vi "criocon.vi"() -> ()   [LabVIEW 2017]
panel:
  in  "Tab Control":enum32{"Page 1", "Page 2"}(tab)
  out "T (K)":dbl=20.57397 format="%6.3f"
  in  "stop":bool
  in  "VISA Resource Name":refnum<visa-resource-name>="GPIB0::12::INSTR"
  in  "wait (ms)":u32=20
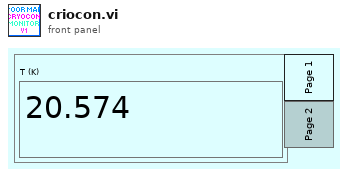
[diagram p1: front panel]
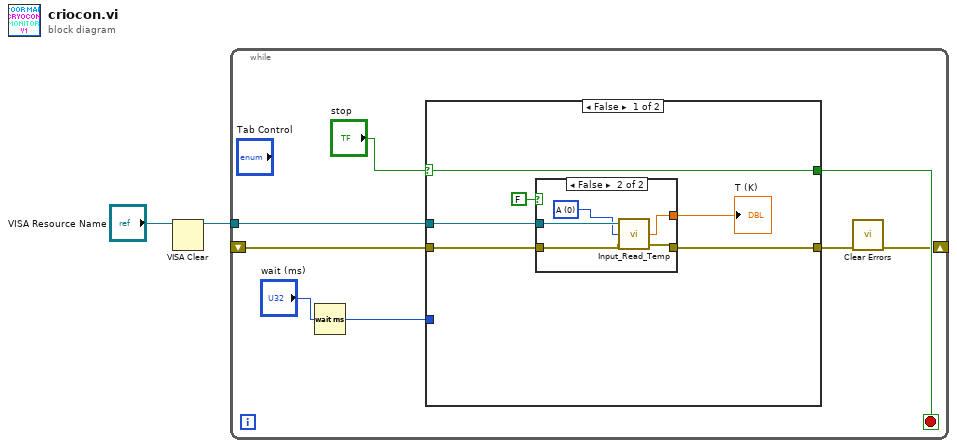
[diagram p0: block diagram]
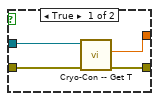
[diagram p2: hidden frame]
diagram:
  n1 = VISA Clear(VISA resource name="VISA Resource Name") -> (VISA resource name out=w1:refnum<visa-resource-name>)  [unwired: 1 in, 1 out]
  n2 = while {
    tunnel: w1 -> [w10]
    shift-right: [w3] -> _
    shift-left: _ -> [w5]
    stop <- w7 stop-if-true
    n3 = Wait (ms)(milliseconds to wait="wait (ms)") -> (millisecond timer value=w9:u32)
    n4 = case shown="False" "stop" {
      selector: "stop" -> [w14 w27]
      tunnel: w10 -> [w15 _]
      tunnel: w9 -> [_ _]
      tunnel: [w14 w27] -> w7
      tunnel: [w13 w26] -> w4
      tunnel: w5 -> [w12 w26]
      frame False {
        n5 = case shown="False" FALSE {
          tunnel: [w20 w25] -> w16
          tunnel: w15 -> [w19 w24]
          tunnel: [w18 w21] -> w13
          tunnel: w12 -> [w17 w22]
          frame True {
            n6 = call "Cryo-Con -- Get T.vi"("error in (no error)"=w17, "VISA Resource Name"=w19) -> ("error out"=w18:errorcluster, "Temperature"=w20:dbl)  [unwired: 6 in, 2 out]
          }
          frame False {
            w23 = u8 0 items=["A", "B"] ("Input")
            n7 = call "Input_Read_Temp.vi"("error in (no error)"=w22, "Input"=w23, "VISA In"=w24) -> ("error out"=w21:errorcluster, "Temperature"=w25:dbl)  [unwired: 1 out]
          }
        }
        "T (K)" <- w16
      }
      frame True {
      }
    }
    n8 = call <vilib>:"Clear Errors.vi"("error in (no error)"=w4) -> ("error out"=w3:errorcluster)  [unwired: 5 in, 1 out]
  }
